vi "Get configuration chain.vi"(8 "error in (no error)":errorcluster, 11 "AOTFBase in":refnum<class "Invivo_AOTF.lvclass">) -> (0 "error out":errorcluster, 1 "class name":string[](array[string]), 2 "configuration chain":variant[](array[variant]), 3 "AOTFBase out":refnum<class "Invivo_AOTF.lvclass">)   [LabVIEW 2012, in "Invivo_AOTF.lvclass"]
doc: "Returns an array of variants containing the configuration clusters of each class in the inheritance chain (lowest child class first), together with an array of all class names in the inheritance chain.\n\nFor classes without configuration cluster, the configuration chain contains empty variants."
uses:
  Invivo_AOTF.lvclass
  <vilib>/Distrio/Murmex/Murmex/Murmex.lvclass
  Invivo_AOTF.lvclass/Invivo_AOTF.ctl
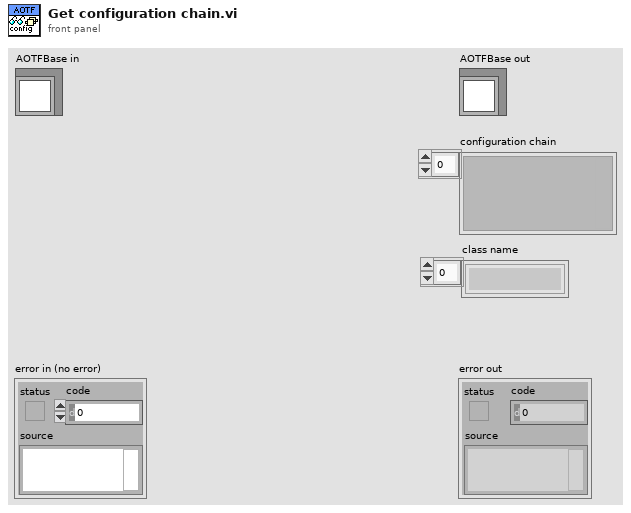
[diagram p1: front panel]
types:
  T1 = typedef "In vivo_AOTF.lvclass/Configuration cluster.ctl" = cluster{"VISA resource name":string, "Baud rate":u32, "Time out":u32, "VISA Wait":dbl[unit], "Power LUT file":path}
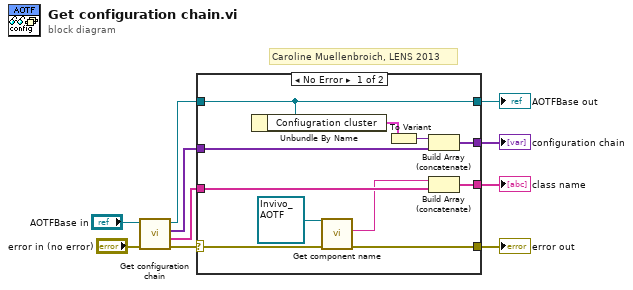
[diagram p0: block diagram]
diagram:
  # "Caroline Muellenbroich, LENS 2013"
  n1 = call-parent "Get configuration chain.vi"("error in (no error)"="error in (no error)", "MurmexBase in"="AOTFBase in") -> ("error out"=w8:errorcluster, "class name"=w6:string[], "configuration chain"=w5:variant[], "MurmexBase out"=w4:refnum<class "Invivo_AOTF.lvclass">)  [unwired: 6 in]
  n2 = case shown="No Error" w8 {
    selector: w8 -> [w21 w22]
    tunnel: [w20 w22] -> w7
    tunnel: w6 -> [w13 w23]
    tunnel: w5 -> [w15 w24]
    tunnel: w4 -> [w18 w25]
    tunnel: [w18 w25] -> w2
    tunnel: [w14 w24] -> w3
    tunnel: [w11 w23] -> w1
    frame No Error {
      n3 = Unbundle By Name(w18) -> ("Confiugration cluster"=w17:T1)
      n4 = call <vilib>:"Get component name.vi"("error in (no error)"=w21, "Murmex in"=refnum<class "Invivo_AOTF.lvclass"> refnum ("AOTF")) -> ("error out"=w20:errorcluster, "component name"=w12:string)  [unwired: 7 in, 1 out]
      n5 = To Variant(anything=w17) -> (Variant=w16:variant)
      n6 = Build Array (concatenate)(w16, w15) -> (w14:variant[])
      n7 = Build Array (concatenate)(w12, w13) -> (w11:string[])
    }
    frame Error {
    }
  }
  "error out" <- w7
  "AOTFBase out" <- w2
  "configuration chain" <- w3
  "class name" <- w1
